vi "GetWaferData.vi"(8 "error in (no error)":errorcluster, 11 "LotData in":refnum<class "LotData.lvclass">) -> (0 "error out":errorcluster, 3 "LotData out":refnum<class "LotData.lvclass">)   [LabVIEW 2012, in "LotData.lvclass"]
uses:
  LotData.lvclass
  Controls/TestData.ctl
  Controls/Measurement.ctl
  <vilib>/addons/database/Auxilliary.llb/DB Tools Parameter Info.ctl
  <vilib>/addons/database/Auxilliary.llb/DB Tools DataTypes.ctl
  <vilib>/addons/database/Auxilliary.llb/DB Tools Parameter Dir.ctl
  LotData.lvclass/LotData.ctl
  Controls/TestArea.ctl
  <vilib>/addons/database/Connection.llb/DB Tools Open Connec (Path).vi
  <vilib>/addons/database/Command.llb/Cmd Set Parameter Value (C).vi
  <vilib>/addons/database/Command.llb/Cmd Execute.vi
  <vilib>/addons/database/Recordset.llb/Rec Fetch Recordset Data (CR).vi
  <vilib>/addons/database/Recordset.llb/Rec Destroy - Command.vi
  <vilib>/addons/database/Command.llb/Cmd Delete.vi
  <vilib>/addons/database/_DB Variant To Data/Database Variant To Data.xnode
  <vilib>/addons/database/NI_Database_API.lvlib
panel:
  out "Array":T1[](array[typedef]) {"50mA Data"."Reverse" format="%#_3g"; "50mA Data"."Current,mA" format="%_6g"; "50mA Data"."Knee Current" format="%#_3g"; "50mA Data"."WL" format="%_6g"; "50mA Data"."Voltage" format="%_6g"; "50mA Data"."Power" format="%_5g"; "20mA Data"."Reverse" format="%#_3g"; "20mA Data"."Current,mA" format="%_6g"; "20mA Data"."Knee Current" format="%#_3g"; "20mA Data"."WL" format="%_6g"; "20mA Data"."Voltage" format="%_6g"; "20mA Data"."Power" format="%_5g"}
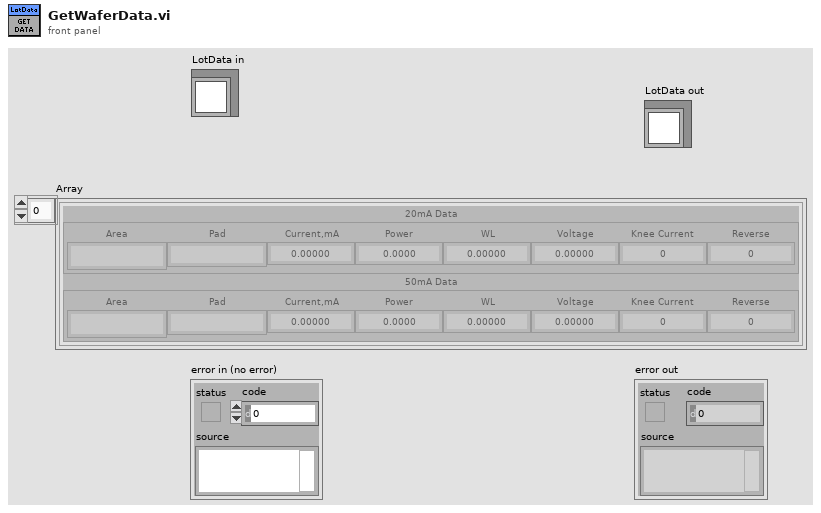
[diagram p1: front panel]
types:
  T1 = typedef "TestData.ctl" = cluster{"20mA Data":T2, "50mA Data ":T2}
  T2 = typedef "Measurement.ctl" = cluster{"Area":string, "Pad":string, "Current,mA":dbl, "Power":dbl, "WL":dbl, "Voltage":dbl, "Knee Current":dbl, "Reverse":dbl}
  T3 = typedef "NI_Database_API.lvlib/DB Tools Parameter Info.ctl" = cluster{"parameter name":string, "type":T4, "direction":T5, "value":variant}
  T4 = typedef "NI_Database_API.lvlib/DB Tools DataTypes.ctl" = enum16{"String", "Long (I32)", "Single (SGL)", "Double (DBL)", "Date/Time", "Binary"}
  T5 = typedef "NI_Database_API.lvlib/DB Tools Parameter Dir.ctl" = enum32{"Input", "Output", "Input/Output", "Return Value"}
  T6 = typedef "TestArea.ctl" = string
  T7 = typedef "NI_Database_API.lvlib/Conn ObjectReference.ctl" = refnum<k1>
  T8 = typedef "NI_Database_API.lvlib/Cmd ObjectReference.ctl" = refnum<k1>
  T9 = typedef "NI_Database_API.lvlib/Cmd-Rec Object Reference.ctl" = refnum<k1>
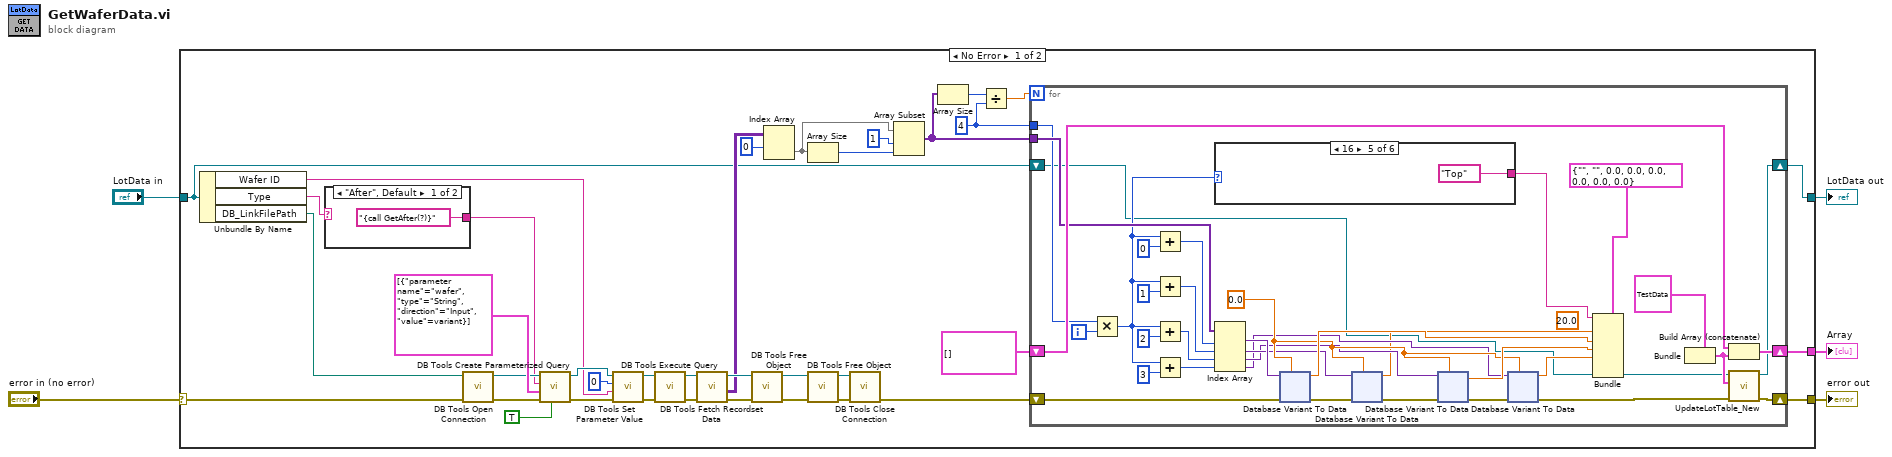
[diagram p0: block diagram]
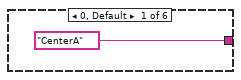
[diagram p2: hidden frame]
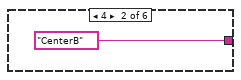
[diagram p3: hidden frame]
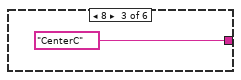
[diagram p4: hidden frame]
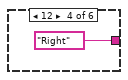
[diagram p5: hidden frame]
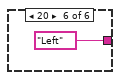
[diagram p6: hidden frame]
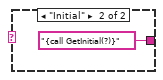
[diagram p7: hidden frame]
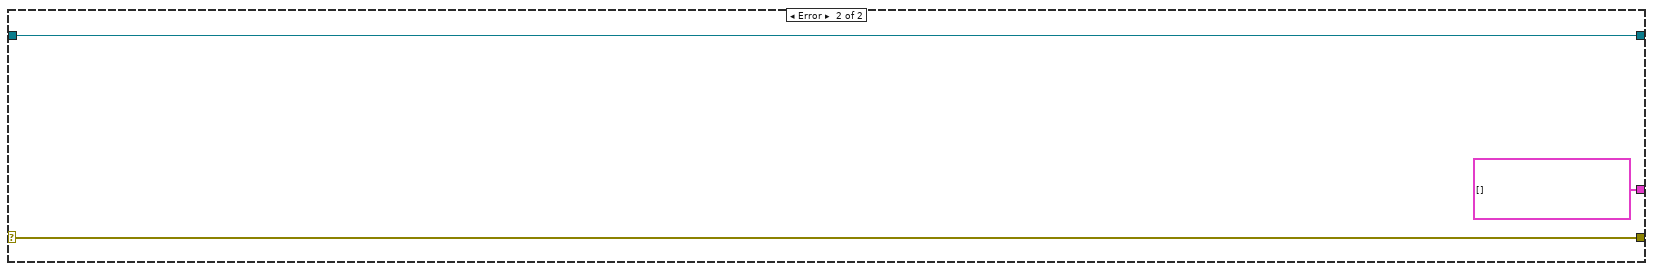
[diagram p8: hidden frame]
diagram:
  n1 = case shown="No Error" "error in (no error)" {
    selector: "error in (no error)" -> [w7 w216]
    tunnel: [w10 w216] -> w2
    tunnel: [w8 w215] -> w1
    tunnel: "LotData in" -> [w9 w215]
    tunnel: [w11 T1[] []] -> w3
    frame No Error {
      w15 = 4 ("y")
      n2 = Unbundle By Name(w9) -> ("Wafer ID"=w13:string, "Type"=w42:string, "DB_LinkFilePath"=w6:path)
      n3 = case shown="\"After\", Default" w42 {
        tunnel: ["{call GetAfter(?)}" ("SQL query") "{call GetInitial(?)}" ("SQL query")] -> w12
        frame "After", Default {
        }
        frame "Initial" {
        }
      }
      n4 = call-poly <vilib>:"DB Tools Open Connection.vi"("error in (no error)"=w7, "connection information"=w6) -> ("error out"=w38:errorcluster, "connection reference"=w39:T7)  [unwired: 6 in]
      n5 = call <vilib>:"DB Tools Create Parameterized Query.vi"("stored procedure? (F)"=TRUE, "error in (no error)"=w38, "parameters"=T3[] [{"parameter name"="wafer", "type"=enum."String", "direction"=enum."Input", "value"=variant}], "SQL query"=w12, "connection reference"=w39) -> ("error out"=w36:errorcluster, "command reference"=w35:T8)  [unwired: 2 in, 1 out]
      n6 = call-poly <vilib>:"DB Tools Set Parameter Value.vi"("error in (no error)"=w36, "value"=w13, "parameter index"=0, "command reference"=w35) -> ("error out"=w32:errorcluster, "command reference out"=w33:T8)  [unwired: 4 in]
      n7 = call-poly <vilib>:"DB Tools Execute Query.vi"("error in (no error)"=w32, "command reference"=w33) -> ("error out"=w27:errorcluster, "command-recordset reference"=w28:T9)  [unwired: 6 in]
      n8 = call-poly <vilib>:"DB Tools Fetch Recordset Data.vi"("error in (no error)"=w27, "command-recordset reference"=w28) -> ("error out"=w26:errorcluster, "recordset data"=w24:variant[][], "command-recordset reference out"=w25:T9)  [unwired: 3 in]
      n9 = call-poly <vilib>:"DB Tools Free Object.vi"("error in (no error)"=w26, "command-recordset reference"=w25) -> ("error out"=w34:errorcluster, "command reference"=w29:T8)  [unwired: 8 in]
      n10 = Index Array(array=w24, index (row)=0) -> (element=w19:variant[])  [unwired: 1 in]
      n11 = Array Size(array=w19) -> (size(s)=w17:i32)
      n12 = call-poly <vilib>:"DB Tools Free Object.vi"("error in (no error)"=w34, "command reference"=w29) -> ("error out"=w30:errorcluster, "connection reference"=w31:T7)  [unwired: 8 in]
      n13 = call <vilib>:"DB Tools Close Connection.vi"("error in (no error)"=w30, "connection reference"=w31) -> ("error out"=w20:errorcluster)  [unwired: 5 in]
      n14 = Array Subset(array=w19, index=1, length=w17) -> (w18:variant[])
      n15 = Array Size(array=w18) -> (size(s)=w16:i32)
      n16 = Divide(x=w16, y=w15) -> (x/y=w14:dbl)
      n17 = for {
        N: w14 -> [_]
        tunnel: w18 -> [w66]
        shift-right: [w75] -> w11
        shift-left: T1[] [] -> [w77]
        shift-right: [w44] -> w10
        shift-left: w20 -> [w54]
        tunnel: w15 -> [w53]
        shift-right: [w46] -> w8
        shift-left: w9 -> [w47]
        i -> [w76]
        (unwired) 20.0 ("Current,mA")
        w67 = 0.0
        n18 = Multiply(x=w53, y=w76) -> (x*y=w51:i32)
        n19 = Add(x=w51, y=0 ("index")) -> (x+y=w65:i32)
        n20 = Add(x=w51, y=1 ("index")) -> (x+y=w64:i32)
        n21 = Add(x=w51, y=2 ("index")) -> (x+y=w63:i32)
        n22 = Add(x=w51, y=3 ("index")) -> (x+y=w62:i32)
        n23 = case shown="16" w51 {
          tunnel: [T6 "CenterA" ("Area") T6 "CenterB" ("Area") T6 "CenterC" ("Area") T6 "Right" ("Area") T6 "Top" ("Area") T6 "Left" ("Area")] -> w50
          frame 0, Default {
          }
          frame 4 {
          }
          frame 8 {
          }
          frame 12 {
          }
          frame 16 {
          }
          frame 20 {
          }
        }
        n24 = Index Array(array=w66, index #1=w65, index #2=w64, index #3=w63, index #4=w62) -> (element #1=w61:variant, element #2=w59:variant, element #3=w58:variant, element #4=w57:variant)
        n25 = xnode "Database Variant To Data"("database variant"=w61, "error in (no error)"=w54, "type"=w67) -> ("data"=w70:dbl, "error out"=w60:errorcluster)
        n26 = xnode "Database Variant To Data"("database variant"=w59, "error in (no error)"=w60, "type"=w67) -> ("data"=w52:dbl, "error out"=w56:errorcluster)
        n27 = xnode "Database Variant To Data"("database variant"=w58, "error in (no error)"=w56, "type"=w67) -> ("data"=w69:dbl, "error out"=w55:errorcluster)
        n28 = xnode "Database Variant To Data"("database variant"=w57, "error in (no error)"=w55, "type"=w67) -> ("data"=w68:dbl, "error out"=w45:errorcluster)
        n29 = Bundle(cluster=T2 {"Area"="", "Pad"="", "Current,mA"=0.0, "Power"=0.0, "WL"=0.0, "Voltage"=0.0, "Knee Current"=0.0, "Reverse"=0.0} ("20mA Data"), "Area"=w50, "Current,mA"=w52, "Power"=w70, "WL"=w69, "Voltage"=w68) -> ()  [unwired: 3 in, 1 out]
        n30 = Bundle(cluster=T1 {"20mA Data"={"Area"="Left", "Pad"="", "Current,mA"=333.0, "Power"=277.2, "WL"=11.8, "Voltage"=6.4, "Knee Current"=0.0, "Reverse"=0.0}, "50mA Data "={"Area"="", "Pad"="", "Current,mA"=0.0, "Power"=0.0, "WL"=0.0, "Voltage"=0.0, "Knee Current"=0.0, "Reverse"=0.0}} ("input cluster")) -> (w48:T1)  [unwired: 2 in]
        n31 = Build Array (concatenate)(w77, w48) -> (w75:T1[])
        n32 = call-dynamic "UpdateLotTable_New.vi"("error in (no error)"=w45, "input cluster"=w48, "LotData in"=w47) -> ("error out"=w44:errorcluster, "LotData out"=w46:refnum<class "LotData.lvclass">)  [unwired: 7 in]
      }
    }
    frame Error {
    }
  }
  "error out" <- w2
  "LotData out" <- w1
  "Array" <- w3
